vi "test_CCDSetAndGetSpeed.vi"(6 "Delay between send and receive [ms]":i32=1000, 7 "Test should pass":bool=TRUE, 8 "error in":errorcluster, 9 "tear down connection":bool=TRUE, 10 "set-up a connection":bool=TRUE, 11 "device selection":enum16{"monochromator", "CCD", "SCD"}(ring)=enum."CCD") -> (0 "error out":errorcluster)   [LabVIEW 2023]
uses:
  <vilib>/addons/_JKI Toolkits/Caraya/classes/Test/Test.lvclass
  <vilib>/addons/_JKI Toolkits/Caraya/classes/Assert/Assert.lvclass
  horiba.test.lvlib
  <vilib>/addons/_JKI Toolkits/Caraya/classes/Assert/Assert Equal Value and Type_Variant.vi
  <vilib>/addons/_JKI Toolkits/Caraya/classes/Assert/Assert Not Error.vi
  <vilib>/addons/_JKI Toolkits/Caraya/classes/Assert/Assert Equal Value_Variant.vi
  Classes/CCD/CCD.lvclass
  Classes/GenericDevice/GenericDevice.lvclass
panel:
  # "Connector Pane"
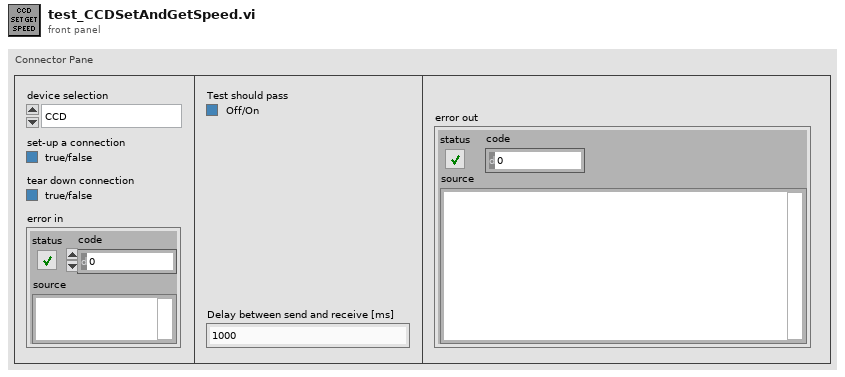
[diagram p1: front panel]
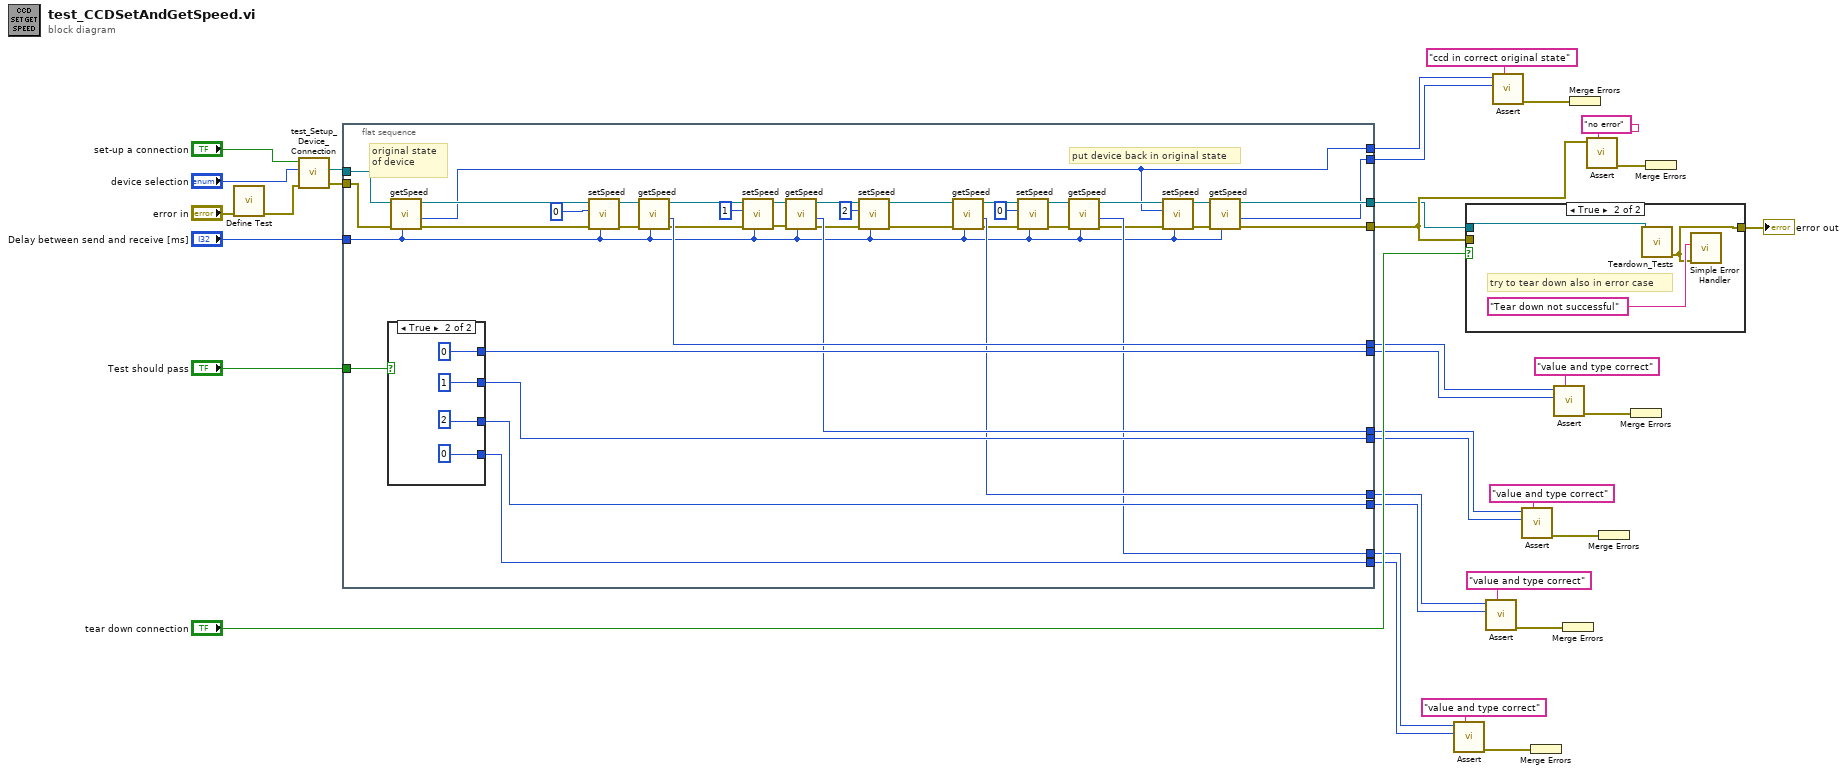
[diagram p0: block diagram]
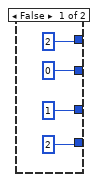
[diagram p2: hidden frame]
diagram:
  n1 = call <vilib>:"Define Test.vi"("error in (no error)"="error in") -> ("error out"=w7:errorcluster)  [unwired: 9 in, 1 out]
  n2 = call "test_Setup_Device_Connection.vi"("error in (no error)"=w7, "device selection"="device selection", "set-up a connection"="set-up a connection") -> ("error out"=w8:errorcluster, "CCD out"=w6:refnum<class "CCD.lvclass">)  [unwired: 5 in, 2 out]
  n3 = flat-sequence {
    tunnel: w8 -> [w68]
    tunnel: w6 -> [w69]
    tunnel: [w51] -> w29
    tunnel: "Test should pass" -> [w74]
    tunnel: [w66] -> w28
    tunnel: [w65] -> w25
    tunnel: [w39] -> w24
    tunnel: [w62] -> w23
    tunnel: [w61] -> w21
    tunnel: [w60] -> w19
    tunnel: [w59] -> w2
    tunnel: [w73] -> w22
    tunnel: [w72] -> w20
    tunnel: [w70] -> w18
    tunnel: [w71] -> w1
    tunnel: "Delay between send and receive [ms]" -> [w40]
    frame #0 {
      # "put device back in original state"
      # "original state of device"
      n4 = case shown="True" w74 {
        tunnel: [2 ("token") 0 ("token")] -> w73
        tunnel: [0 ("token") 1 ("token")] -> w72
        tunnel: [1 ("token") 2 ("token")] -> w70
        tunnel: [2 ("token") 0 ("token")] -> w71
        frame False {
        }
        frame True {
        }
      }
      n5 = call "getSpeed.vi"("Delay between send and receive [ms]"=w40, "error in (no error)"=w68, "CCD in"=w69) -> ("error out"=w41:errorcluster, "token"=w39:i32, "CCD out"=w57:refnum<class "CCD.lvclass">)  [unwired: 5 in, 1 out]
      n6 = call "setSpeed.vi"("Delay between send and receive [ms]"=w40, "error in (no error)"=w41, "token"=0, "CCD in"=w57) -> ("error out"=w42:errorcluster, "CCD out"=w63:refnum<class "CCD.lvclass">)  [unwired: 4 in, 2 out]
      n7 = call "getSpeed.vi"("Delay between send and receive [ms]"=w40, "error in (no error)"=w42, "CCD in"=w63) -> ("error out"=w43:errorcluster, "token"=w62:i32, "CCD out"=w64:refnum<class "CCD.lvclass">)  [unwired: 5 in, 1 out]
      n8 = call "setSpeed.vi"("Delay between send and receive [ms]"=w40, "error in (no error)"=w43, "token"=1, "CCD in"=w64) -> ("error out"=w44:errorcluster, "CCD out"=w52:refnum<class "CCD.lvclass">)  [unwired: 4 in, 2 out]
      n9 = call "getSpeed.vi"("Delay between send and receive [ms]"=w40, "error in (no error)"=w44, "CCD in"=w52) -> ("error out"=w45:errorcluster, "token"=w61:i32, "CCD out"=w56:refnum<class "CCD.lvclass">)  [unwired: 5 in, 1 out]
      n10 = call "setSpeed.vi"("Delay between send and receive [ms]"=w40, "error in (no error)"=w45, "token"=2, "CCD in"=w56) -> ("error out"=w46:errorcluster, "CCD out"=w55:refnum<class "CCD.lvclass">)  [unwired: 4 in, 2 out]
      n11 = call "getSpeed.vi"("Delay between send and receive [ms]"=w40, "error in (no error)"=w46, "CCD in"=w55) -> ("error out"=w47:errorcluster, "token"=w60:i32, "CCD out"=w54:refnum<class "CCD.lvclass">)  [unwired: 5 in, 1 out]
      n12 = call "setSpeed.vi"("Delay between send and receive [ms]"=w40, "error in (no error)"=w47, "token"=0, "CCD in"=w54) -> ("error out"=w48:errorcluster, "CCD out"=w53:refnum<class "CCD.lvclass">)  [unwired: 4 in, 2 out]
      n13 = call "getSpeed.vi"("Delay between send and receive [ms]"=w40, "error in (no error)"=w48, "CCD in"=w53) -> ("error out"=w49:errorcluster, "token"=w59:i32, "CCD out"=w58:refnum<class "CCD.lvclass">)  [unwired: 5 in, 1 out]
      n14 = call "setSpeed.vi"("Delay between send and receive [ms]"=w40, "error in (no error)"=w49, "token"=w39, "CCD in"=w58) -> ("error out"=w50:errorcluster, "CCD out"=w67:refnum<class "CCD.lvclass">)  [unwired: 4 in, 2 out]
      n15 = call "getSpeed.vi"("Delay between send and receive [ms]"=w40, "error in (no error)"=w50, "CCD in"=w67) -> ("error out"=w51:errorcluster, "token"=w65:i32, "CCD out"=w66:refnum<class "CCD.lvclass">)  [unwired: 5 in, 1 out]
    }
  }
  n16 = call-poly <vilib>:"Assert.vi"("Label"="value and type correct" ("Label (VI Title)"), "Y"=w1, "X"=w2) -> ("error out"=w11:errorcluster)  [unwired: 7 in, 1 out]
  n17 = case shown="True" "tear down connection" {
    tunnel: w28 -> [_ w85]
    tunnel: [w83 w84] -> w9
    tunnel: w29 -> [w83 _]
    frame False {
    }
    frame True {
      # "try to tear down also in error case"
      n18 = call "Teardown_Tests.vi"("horiba.lvlib:GenericDevice"=w85) -> ("error out"=w84:errorcluster)  [unwired: 9 in, 1 out]
      n19 = call <vilib>:"Simple Error Handler.vi"("error source (\" \")"="Tear down not successful" ("error source (\" \")"), "error in (no error)"=w84) -> ()  [unwired: 3 in, 5 out]
    }
  }
  "error out" <- w9
  n20 = call-poly <vilib>:"Assert.vi"("Label"="value and type correct" ("Label (VI Title)"), "Y"=w18, "X"=w19) -> ("error out"=w10:errorcluster)  [unwired: 7 in, 1 out]
  n21 = call-poly <vilib>:"Assert.vi"("Label"="ccd in correct original state" ("Label (VI Title)"), "Y"=w25, "X"=w24) -> ("error out"=w27:errorcluster)  [unwired: 7 in, 1 out]
  n22 = call-poly <vilib>:"Assert.vi"("Label"="value and type correct" ("Label (VI Title)"), "Y"=w20, "X"=w21) -> ("error out"=w14:errorcluster)  [unwired: 7 in, 1 out]
  n23 = Merge Errors(w11) -> ()  [unwired: 1 out]
  n24 = call-poly <vilib>:"Assert.vi"("Label"="value and type correct" ("Label (VI Title)"), "Y"=w22, "X"=w23) -> ("error out"=w16:errorcluster)  [unwired: 7 in, 1 out]
  n25 = Merge Errors(w10) -> ()  [unwired: 1 out]
  n26 = Merge Errors(w27) -> ()  [unwired: 1 out]
  n27 = call-poly <vilib>:"Assert.vi"("Label"="no error" ("Label (VI Title)"), "Not Error?"=w29) -> ("error out"=w31:errorcluster)  [unwired: 8 in, 1 out]
  n28 = Merge Errors(w14) -> ()  [unwired: 1 out]
  n29 = Merge Errors(w16) -> ()  [unwired: 1 out]
  n30 = Merge Errors(w31) -> ()  [unwired: 1 out]
